vi "Close Config File.vi"(8 "error in (no error)":errorcluster, 10 "refnum":T1, 11 "Process in":refnum<class "Process.lvclass">) -> (0 "error out":errorcluster, 2 "file path":path, 3 "Process out":refnum<class "Process.lvclass">)   [LabVIEW 2020, in "Configuration File.lvlib"]
doc: "High-level function for opening configuration file data from Process class."
uses:
  Configuration File.lvlib
  User Interface/Process/Process.lvclass
  <vilib>/Utility/config.llb/Config Data RefNum.ctl
  <vilib>/Utility/config.llb/NI_LVConfig.lvlib
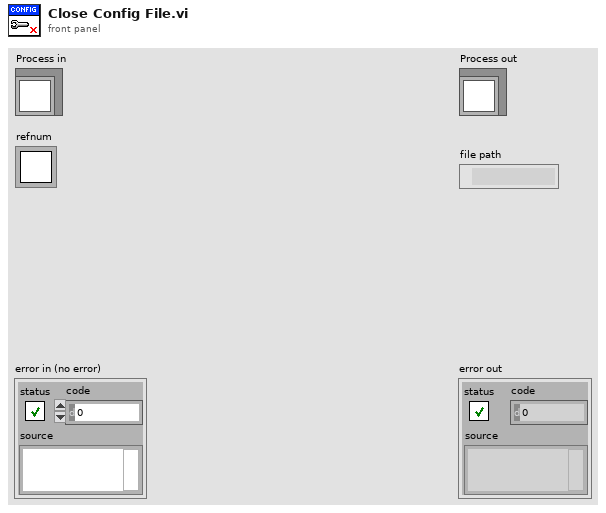
[diagram p1: front panel]
types:
  T1 = typedef "NI_LVConfig.lvlib/Config Data RefNum.ctl" = refnum<k1>
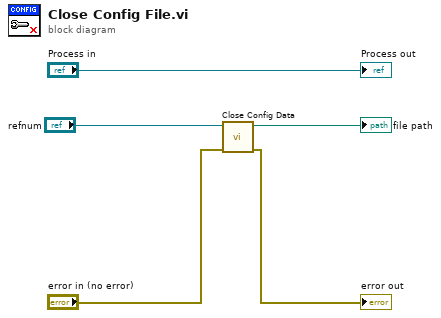
[diagram p0: block diagram]
diagram:
  n1 = call <vilib>:"Close Config Data.vi"("error in (no error)"="error in (no error)", "refnum"="refnum") -> ("error out"=→"error out":errorcluster, "file path"=→"file path":path)  [unwired: 8 in]
  "Process out" <- "Process in"
